vi "Build Mission Array.vi"(8 "Error In":errorcluster) -> (0 "Error Out":errorcluster, 3 "Number of Waypoints":i32)   [LabVIEW 2014]
uses:
  Controls/Mission Planning Controls/MAVLINK Mission Item.ctl
  Controls/MAVLINK Mav Frame.ctl
  Aircraft Information/Sub VI/Selected Aircraft/SubVI/Get Selected Aircraft.vi
  Commands/Mission Planning/MISSION_ITEM SubVI/MISSION_ITEM Set ROI.vi
  Missions/FGVs/Virtual Waypoints/Methods/Get Selected Virtual WP.vi
  Aircraft Information/Sub VI/Get Aircraft GPS.vi
  Commands/Mission Planning/MISSION_ITEM SubVI/MISSION_ITEM Land.vi
  Commands/Mission Planning/MISSION_ITEM SubVI/MISSION_ITEM Loiter (Time).vi
  Commands/Mission Planning/MISSION_ITEM SubVI/MISSION_ITEM Takeoff.vi
  Missions/FGVs/Virtual Waypoints/Methods/Get Virtual Waypoints.vi
  Commands/Mission Planning/MISSION_ITEM SubVI/MISSION_ITEM Change Speed.vi
  Commands/Mission Planning/MISSION_ITEM SubVI/MISSION_ITEM Waypoint.vi
  Aircraft Information/Sub VI/Set Aircraft Waypoints.vi
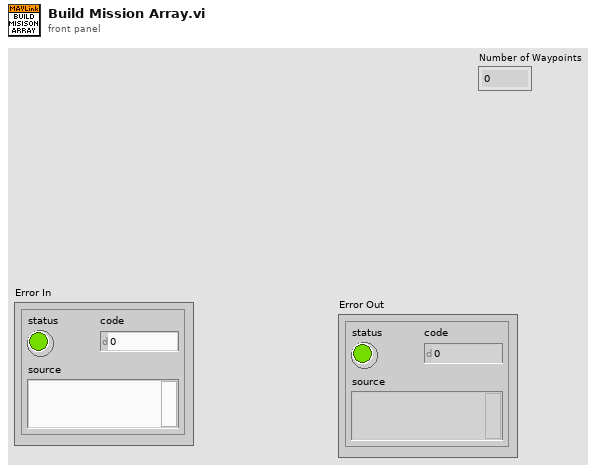
[diagram p1: front panel]
types:
  T1 = typedef "MAVLINK Mission Item.ctl" = cluster{"target_system":u8, "target_component":u8, "sequence":u16, "frame":T2, "command":u16, "current":bool, "autocontinue":bool, "param1":sgl, "param2":sgl, "param3":sgl, "param4":sgl, "Lat":sgl, "Lon":sgl, "Altitude (m)":sgl}
  T2 = typedef "MAVLINK Mav Frame.ctl" = enum8{"GLOBAL", "LOCAL NED", "MISSION", "GLOBAL RELATIVE ALT", "LOCAL ENU", "GLOBAL INT", "GLOBAL RELATIVE ALT INT", "LOCAL OFFSET NED", "BODY NED", "BODY OFFSET NED", "GLOBAL TERRAIN ALT", "GLOBAL TERRAIN ALT INT"}
  T3 = typedef "Virtual Waypoint.ctl" = cluster{"Waypoint Type":T4, "Lat":sgl, "Lon":sgl, "Altitude (m)":sgl, "Inspection Height (m)":sgl, "Circumnavigate Radius (m)":sgl, "Grid Waypoint?":bool, "Capture Photo":bool, "Speed (m/s)":sgl}
  T4 = typedef "Waypoint Type.ctl" = enum16{"PASS-THROUGH", "INSPECT", "CIRCUMNAVIGATE"}
  T5 = typedef "Aircraft GPS Data.ctl" = cluster{"Latitude (degrees)":dbl, "Longitude (degrees)":dbl, "Altitude (m)":dbl, "Fix Type":T6, "HDOP (cm)":u16, "VDOP (cm)":u16, "Ground Speed (m/s)":dbl, "Coarse Over Ground (degrees)":u16, "Number of Satellites":u8}
  T6 = typedef "GPS Fix Type.ctl" = enum16{"No Fix 0", "No Fix 1", "2D Fix", "3D Fix", "DGPS", "RTK"}
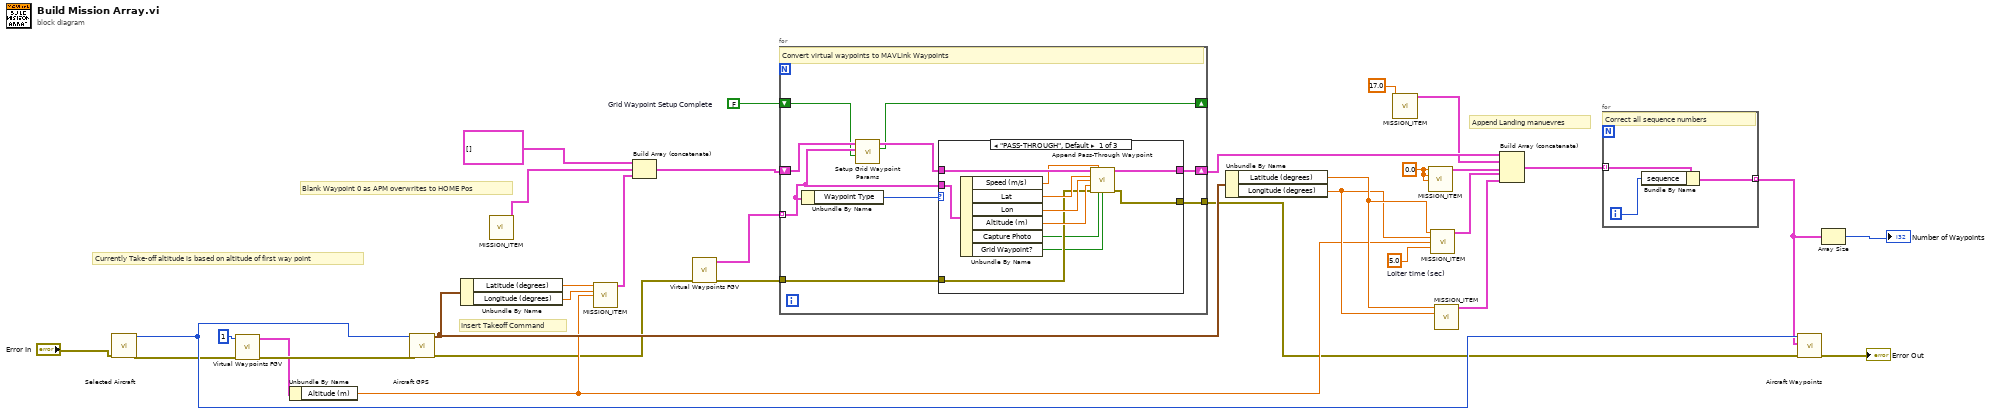
[diagram p0: block diagram]
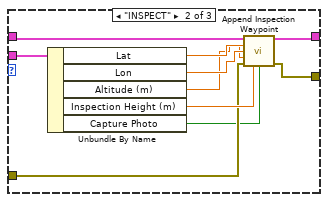
[diagram p2: hidden frame]
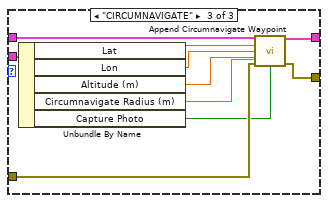
[diagram p3: hidden frame]
diagram:
  w1 = FALSE  # Grid Waypoint Setup Complete
  w17 = sgl 0.0 ("Lat")
  w28 = sgl 5.0  # Loiter time (sec)
  # "Currently Take-off altitude is based on altitude of first way point"
  # "Append Landing manuevres"
  # "Insert Takeoff Command"
  # "Blank Waypoint 0 as APM overwrites to HOME Pos"
  n1 = call-poly "Selected Aircraft.vi"("Error In"="Error In") -> ("Error Out"=w9:errorcluster, "Selected Aircraft ID Out"=w23:u8)  [unwired: 9 in]
  n2 = call-poly "Virtual Waypoints FGV.vi"("Error In"=w9, "Waypoint Number"=1) -> ("Error Out"=w12:errorcluster, "Virtual Waypoint out"=w11:T3)  [unwired: 8 in]
  n3 = Unbundle By Name(w11) -> ("Altitude (m)"=w14:sgl)
  n4 = call-poly "Aircraft GPS.vi"("Error In"=w12, "Aircraft ID"=w23) -> ("Error Out"=w8:errorcluster, "Aircraft GPS Data Out"=w27:T5)  [unwired: 8 in]
  n5 = Unbundle By Name(w27) -> ("Latitude (degrees)"=w31:dbl, "Longitude (degrees)"=w30:dbl)
  n6 = call-poly "MISSION_ITEM.vi"() -> ("Mission Item"=w32:T1)  [unwired: 15 in]
  n7 = call-poly "MISSION_ITEM.vi"("Lat"=w31, "Lon"=w30, "Altitude (m)"=w14) -> ("Mission Item"=w29:T1)  [unwired: 12 in]
  n8 = Build Array (concatenate)(T1[] [] ("array"), w32, w29) -> (w13:T1[])
  n9 = call-poly "Virtual Waypoints FGV.vi"("Error In"=w8) -> ("Error Out"=w7:errorcluster, "Virtual Waypoints Out"=w6:T3[])  [unwired: 9 in]
  n10 = for {
    shift-right: [w40] -> w4
    shift-left: w13 -> [w38]
    tunnel: w7 -> [w41]
    tunnel: w6 -> [w36] mode=indexing
    tunnel: [w39] -> w5
    shift-right: [w34] -> _
    shift-left: w1 -> [w35]
    # "Convert virtual waypoints to MAVLink Waypoints"
    n11 = Unbundle By Name(w36) -> ("Waypoint Type"=w42:T4)
    n12 = call "Setup Grid Waypoint Params.vi"("Grid Setup Complete?"=w35, "Virtual Waypoint"=w36, "Waypoints"=w38) -> ("Grid Setup Complete? Out"=w34:bool, "Waypoints Out"=w37:T1[])  [unwired: 7 in]
    n13 = case shown="\"PASS-THROUGH\", Default" w42 {
      tunnel: w36 -> [w52 w63 w71]
      tunnel: w37 -> [w53 w62 w70]
      tunnel: w41 -> [w48 w57 w65]
      tunnel: [w47 w55 w73] -> w40
      tunnel: [w46 w56 w72] -> w39
      frame "PASS-THROUGH", Default {
        n14 = Unbundle By Name(w52) -> ("Speed (m/s)"=w43:sgl, "Lat"=w51:sgl, "Lon"=w50:sgl, "Altitude (m)"=w49:sgl, "Capture Photo"=w45:bool, "Grid Waypoint?"=w44:bool)
        n15 = call "Append Pass-Through Waypoint.vi"("Waypoint Array In"=w53, "Speed (m/s)"=w43, "Lat"=w51, "Lon"=w50, "Altitude (m)"=w49, "Error In"=w48, "Capture Photo"=w45, "Grid Waypoint?"=w44) -> ("appended array"=w47:T1[], "Error Out"=w46:errorcluster)  [unwired: 6 in]
      }
      frame "INSPECT" {
        n16 = Unbundle By Name(w63) -> ("Lat"=w61:sgl, "Lon"=w60:sgl, "Altitude (m)"=w59:sgl, "Inspection Height (m)"=w58:sgl, "Capture Photo"=w54:bool)
        n17 = call "Append Inspection Waypoint.vi"("Waypoint Array In"=w62, "Lat"=w61, "Lon"=w60, "Altitude (m)"=w59, "Error In"=w57, "Inspection altitude (m)"=w58, "Capture Photo"=w54) -> ("appended array"=w55:T1[], "Error Out"=w56:errorcluster)  [unwired: 7 in]
      }
      frame "CIRCUMNAVIGATE" {
        n18 = Unbundle By Name(w71) -> ("Lat"=w69:sgl, "Lon"=w68:sgl, "Altitude (m)"=w67:sgl, "Circumnavigate Radius (m)"=w66:sgl, "Capture Photo"=w64:bool)
        n19 = call "Append Circumnavigate Waypoint.vi"("Waypoint Array In"=w70, "Lat"=w69, "Lon"=w68, "Altitude (m)"=w67, "Error In"=w65, "Circumnavigate radius (m)"=w66, "Capture Photo"=w64) -> ("appended array"=w73:T1[], "Error Out"=w72:errorcluster)  [unwired: 7 in]
      }
    }
  }
  n20 = Unbundle By Name(w27) -> ("Latitude (degrees)"=w25:dbl, "Longitude (degrees)"=w18:dbl)
  n21 = call-poly "MISSION_ITEM.vi"("Speed (m/s)"=sgl 17.0) -> ("Mission Item"=w3:T1)  [unwired: 14 in]
  n22 = call-poly "MISSION_ITEM.vi"("Lat"=w17, "Lon"=w17, "Altitude (m)"=w17) -> ("Mission Item"=w16:T1)  [unwired: 12 in]
  n23 = call-poly "MISSION_ITEM.vi"("Lat"=w25, "Lon"=w18, "Altitude (m)"=w14, "Loiter time (sec)"=w28) -> ("Mission Item"=w26:T1)  [unwired: 11 in]
  n24 = call-poly "MISSION_ITEM.vi"("Lat"=w25, "Lon"=w18) -> ("Mission Item"=w24:T1)  [unwired: 13 in]
  n25 = Build Array (concatenate)(w4, w3, w16, w26, w24) -> (w21:T1[])
  n26 = for {
    tunnel: w21 -> [w76] mode=indexing
    tunnel: [w74] -> w20 mode=indexing
    i -> [w75]
    # "Correct all sequence numbers"
    n27 = Bundle By Name(cluster=w76, "sequence"=w75) -> (w74:T1)
  }
  n28 = call-poly "Aircraft Waypoints.vi"("Error In"=w5, "Waypoints In"=w20, "Aircraft ID"=w23) -> ("Error Out"=→"Error Out":errorcluster)  [unwired: 8 in]
  n29 = Array Size(array=w20) -> (size(s)=→"Number of Waypoints":i32)
